vi "Blockage Correction.vi"() -> ()   [LabVIEW 2017]
panel:
  out "Collector Blockage Correction (Ec)":dbl
  out "Jet-Deflection Correction (Es)":dbl
  out "Nozzle Blockage Correction (En)":dbl
  in  "Test Section Length (Lts)":dbl
  in  "Equivalent Collector Radius (Rc)":dbl
  in  "Measured Drag Coeff. (Cdm)":dbl
  in  "Collector Area (Ac)":dbl
  in  "Equivalent Nozzle Radius (Rn)":dbl
  in  "Turn-table Centre (Xm)":dbl
  in  "Nozzle Area (An)":dbl=0.667
  in  "Vehicle Frontal Area (Am)":dbl
  in  "Vehicle Length (Lm)":dbl
  in  "Vehicle Volume (Vm)":dbl
  in  "Tunnel Shape Factor (t)":dbl=0.62
  # "Ref: SAE 960671"
  # "Output Corrections"
  # "Input Parameters"
  # "Open-Jet Blockage Correction"
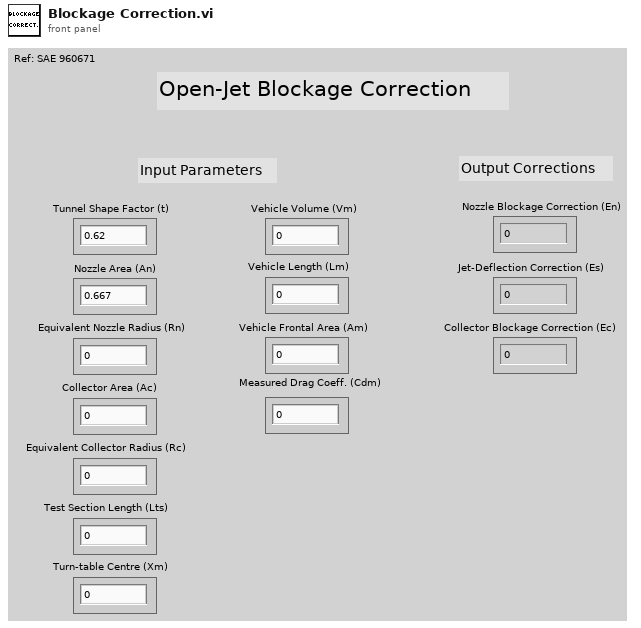
[diagram p1: front panel]
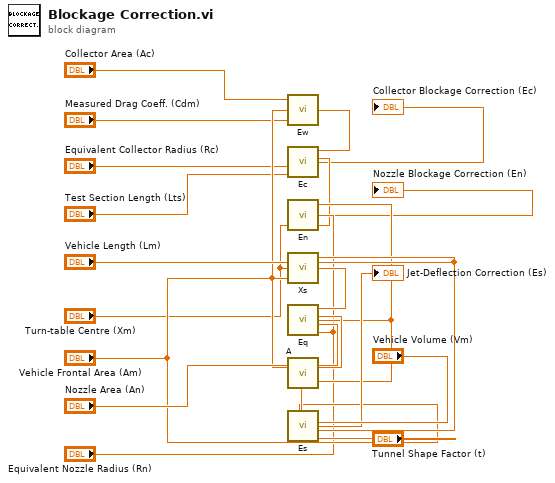
[diagram p0: block diagram]
diagram:
  n1 = call "Ew.vi"("Measured Drag Coeff. (Cdm)"="Measured Drag Coeff. (Cdm)", "Vehicle Frontal Area (Am)"="Vehicle Frontal Area (Am)", "Collector Area (Ac)"="Collector Area (Ac)") -> ("Wake Blockage Factor (Ew)"=w8:dbl)
  n2 = call "Ec.vi"("Test Section Length (Lts)"="Test Section Length (Lts)", "Equivalent Collector Radius (Rc)"="Equivalent Collector Radius (Rc)", "Turn-table Centre (Xm)"="Turn-table Centre (Xm)", "Wake Blockage Factor (Ew)"=w8) -> ("Collector Blockage Correction (Ec)"=→"Collector Blockage Correction (Ec)":dbl)
  n3 = call "Xs.vi"("Vehicle Frontal Area (Am)"="Vehicle Frontal Area (Am)", "Turn-table Centre (Xm)"="Turn-table Centre (Xm)", "Vehicle Length (Lm)"="Vehicle Length (Lm)") -> ("Nozzle-source point (Xs)"=w18:dbl)
  n4 = call "Eq.vi"("Equivalent Nozzle Radius (Rn)"="Equivalent Nozzle Radius (Rn)", "Nozzle Area (An)"="Nozzle Area (An)", "Vehicle Frontal Area (Am)"="Vehicle Frontal Area (Am)", "Nozzle-source point (Xs)"=w18) -> ("Nozzle Blockage Factor (Eq)"=w5:dbl)
  n5 = call "En.vi"("Turn-table Centre (Xm)"="Turn-table Centre (Xm)", "Equivalent Nozzle Radius (Rn)"="Equivalent Nozzle Radius (Rn)", "Nozzle Blockage Factor (Eq)"=w5) -> ("Nozzle Blockage Correction (En)"=→"Nozzle Blockage Correction (En)":dbl)
  n6 = call "A.vi"("Nozzle Blockage Factor (Eq)"=w5, "Nozzle Area (An)"="Nozzle Area (An)") -> ("Reduced Nozzle (A*)"=w13:dbl)
  n7 = call "Es.vi"("Reduced Nozzle (A*)"=w13, "Vehicle Volume (Vm)"="Vehicle Volume (Vm)", "Vehicle Length (Lm)"="Vehicle Length (Lm)", "Tunnel Shape Factor (t)"="Tunnel Shape Factor (t)", "Vehicle Frontal Area (Am)"="Vehicle Frontal Area (Am)") -> ("Induced Velocity due to Jet Expansion (Es)"=→"Jet-Deflection Correction (Es)":dbl)
